vi "Cannon Logic.vi"() -> ()   [LabVIEW 2019]
uses:
  <vilib>/Rock Robotics/WPI/Solenoid/WPI_SolenoidValue.ctl
  <vilib>/Rock Robotics/WPI/ThirdParty/Phoenix-LabVIEW/Motor Controller/Controls/CTRE_Phoenix_MotorControl_ControlMode.ctl
  <vilib>/Rock Robotics/Network Tables/NT Read Boolean.vi
  Robot Global Data.vi
  <vilib>/Rock Robotics/Network Tables/NT Write Number.vi
  <vilib>/Rock Robotics/WPI/Solenoid/WPI_SolenoidSetEnum.vi
panel:
  out "ballcount":i16
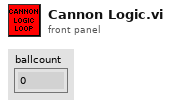
[diagram p1: front panel]
types:
  T1 = typedef "WPI_SolenoidDevRef.ctl" = cluster{"DevStatus":errorcluster, "Pneumatics Control Module":u8, "Forward Solenoid Channel":T2, "Reverse Solenoid Channel":T2}
  T2 = typedef "WPI_SolenoidChannel.ctl" = enum8{"Solenoid 0", "Solenoid 1", "Solenoid 2", "Solenoid 3", "Solenoid 4", "Solenoid 5", "Solenoid 6", "Solenoid 7", "Invalid"}
  T3 = typedef "WPI_MotorControlDeviceRef.ctl" = cluster{"DeviceStatus":errorcluster, "Type":T4, "PWM":cluster{"PWM Channel":T5, "DeadBand":T6}, "CAN":cluster{"Device Number":u8, "SetOutput VI Ref":variant, "GetOutput VI Ref":variant, "Enable VI Ref":variant, "Disable VI Ref":variant, "Data":variant}, "Invert":bool, "DIO PWM":cluster{"PWM \"Enable\" Channel":T5, "DIOChannel":T7, "PWM Rate":dbl}}
  T4 = typedef "WPI_MotorControlType.ctl" = enum16{"PWM", "CAN", "DIO PWM"}
  T5 = typedef "FPGA_DIOPWMChannel.ctl" = enum8{"PWM 0", "PWM 1", "PWM 2", "PWM 3", "PWM 4", "PWM 5", "PWM 6", "PWM 7", "PWM 8", "PWM 9", "PWM MXP 0", "PWM MXP 1", "PWM MXP 2", "PWM MXP 3", "PWM MXP 4", "PWM MXP 5", "PWM MXP 6", "PWM MXP 7", "PWM MXP 8", "PWM MXP 9", "Invalid"}
  T6 = typedef "WPI_PWMDeadband.ctl" = cluster{"Name":string, "maxPositivePwm":i32, "minPositivePwm":i32, "centerPwm":i32, "maxNegativePwm":i32, "minNegativePwm":i32, "angularRange":u16}
  T7 = typedef "FPGA_DIOChannel.ctl" = enum8{"DIO 0", "DIO 1", "DIO 2", "DIO 3", "DIO 4", "DIO 5", "DIO 6", "DIO 7", "DIO 8", "DIO 9", "DIO MXP 0", "DIO MXP 1", "DIO MXP 2", "DIO MXP 3", "DIO MXP 4", "DIO MXP 5", "DIO MXP 6", "DIO MXP 7", "DIO MXP 8", "DIO MXP 9", "DIO MXP 10", "DIO MXP 11", "DIO MXP 12", "DIO MXP 13", "DIO MXP 14", "DIO MXP 15", "SPI Port CS1", "SPI Port CS2", "SPI Port CS3", "SPI Port MISO", "SPI Port MOSI", "Invalid"}
  T8 = typedef "WPI_AnalogChannelDevRef.ctl" = cluster{"DevStatus":errorcluster, "Analog Channel":T9}
  T9 = typedef "FPGA_AIChannel.ctl" = enum8{"AI 0", "AI 1", "AI 2", "AI 3", "AI MXP 0", "AI MXP 1", "AI MXP 2", "AI MXP 3", "Invalid"}
  T10 = typedef "WPI_EncoderDevRef.ctl" = cluster{"DevStatus":errorcluster, "EncoderIndex":T11, "CounterIndex":T12, "DistancePerCount":dbl, "Decoding Type":T13}
  T11 = typedef "FPGA_EncoderIdx.ctl" = enum8{"Enc 0", "Enc 1", "Enc 2", "Enc 3", "Enc 4", "Enc 5", "Enc 6", "Enc 7", "Invalid"}
  T12 = typedef "FPGA_CounterCtrSystemIndex.ctl" = enum8{"Ctr 0", "Ctr 1", "Ctr 2", "Ctr 3", "Ctr 4", "Ctr 5", "Ctr 6", "Ctr 7", "Invalid"}
  T13 = typedef "WPI_EncoderType.ctl" = enum16{"1x", "2x", "4x"}
  T14 = typedef "WPI_SolenoidValue.ctl" = enum16{"Off", "On", "Forward", "Reverse"}
  T15 = typedef "CTRE_Phoenix_MotorControl_ControlMode.ctl" = u16
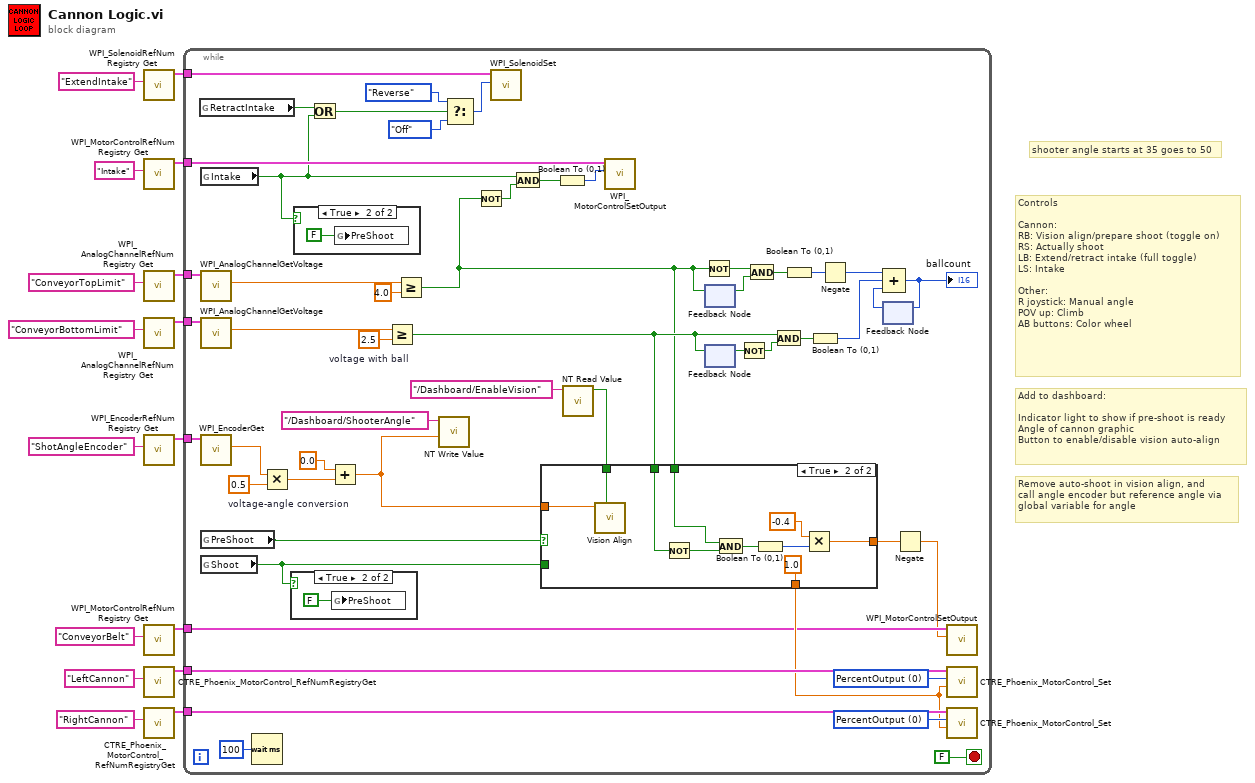
[diagram p0: block diagram]
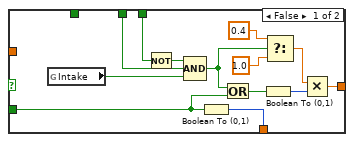
[diagram p4: hidden frame]
diagram:
  # "shooter angle starts at 35 goes to 50"
  # "Remove auto-shoot in vision align, and\ncall angle encoder but reference angle via\nglobal variable for angle"
  # "Add to dashboard:\n\nIndicator light to show if pre-shoot is ready\nAngle of cannon graphic\nButton to enable/disable vision auto-align"
  # "Controls\n\nCannon:\nRB: Vision align/prepare shoot (toggle on)\nRS: Actually shoot\nLB: Extend/retract intake (full toggle)\nLS: Intake\n\nOther:\nR joystick: Manual angle\nPOV up: Climb\nAB buttons: Color wheel"
  n1 = call <vilib>:"WPI_SolenoidRefNum Registry Get.vi"("refnum name"="ExtendIntake") -> ("SolenoidDevRef"=w10:T1)  [unwired: 9 in, 1 out]
  n2 = call <vilib>:"WPI_MotorControlRefNum Registry Get.vi"("refnum name"="Intake") -> ("MotorControlDevRef"=w9:T3)  [unwired: 9 in, 1 out]
  n3 = call <vilib>:"WPI_AnalogChannelRefNum Registry Get.vi"("refnum name"="ConveyorTopLimit") -> ("AIDeviceRef"=w6:T8)  [unwired: 9 in, 1 out]
  n4 = call <vilib>:"WPI_AnalogChannelRefNum Registry Get.vi"("refnum name"="ConveyorBottomLimit") -> ("AIDeviceRef"=w7:T8)  [unwired: 9 in, 1 out]
  n5 = call <vilib>:"WPI_EncoderRefNum Registry Get.vi"("refnum name"="ShotAngleEncoder") -> ("EncoderDevRef"=w1:T10)  [unwired: 9 in, 1 out]
  n6 = call <vilib>:"WPI_MotorControlRefNum Registry Get.vi"("refnum name"="ConveyorBelt") -> ("MotorControlDevRef"=w5:T3)  [unwired: 9 in, 1 out]
  n7 = call <vilib>:"CTRE_Phoenix_MotorControl_RefNumRegistryGet.vi"("refnum name"="LeftCannon") -> ("PhoenixMotorControlDevRef"=w3:T3)  [unwired: 9 in, 1 out]
  n8 = call <vilib>:"CTRE_Phoenix_MotorControl_RefNumRegistryGet.vi"("refnum name"="RightCannon") -> ("PhoenixMotorControlDevRef"=w8:T3)  [unwired: 9 in, 1 out]
  n9 = while {
    tunnel: w10 -> [w63]
    tunnel: w9 -> [w49]
    tunnel: w8 -> [w61]
    tunnel: w7 -> [w60]
    tunnel: w6 -> [w59]
    tunnel: w5 -> [w48]
    tunnel: w3 -> [w55]
    tunnel: w1 -> [w21]
    stop <- FALSE stop-if-true
    w22 = 0.5  # voltage-angle conversion
    w56 = T15 0 items=["PercentOutput"=0, "Position"=1, "Velocity"=2, "Current"=3, "Follower"=5, "MotionProfile"=6, "MotionMagic"=7, "MotionProfileArc"=10, "Disabled"=15] ("Control Mode")
    w54 = T15 0 items=["PercentOutput"=0, "Position"=1, "Velocity"=2, "Current"=3, "Follower"=5, "MotionProfile"=6, "MotionMagic"=7, "MotionProfileArc"=10, "Disabled"=15] ("Control Mode")
    w57 = 2.5  # voltage with ball
    n10 = global read "Robot Global Data.vi" "RetractIntake"() -> (w35:bool)
    n11 = global read "Robot Global Data.vi" "Intake"() -> (w28:bool)
    n12 = call <vilib>:"WPI_AnalogChannelGetVoltage.vi"("AIDeviceRef"=w59) -> ("Voltage"=w30:dbl)  [unwired: 8 in, 2 out]
    n13 = call <vilib>:"WPI_AnalogChannelGetVoltage.vi"("AIDeviceRef"=w60) -> ("Voltage"=w29:dbl)  [unwired: 8 in, 2 out]
    n14 = call <vilib>:"WPI_EncoderGet.vi"("EncoderDevRef"=w21) -> ("Distance"=w23:dbl)  [unwired: 5 in, 5 out]
    n15 = global read "Robot Global Data.vi" "PreShoot"() -> (w33:bool)
    n16 = global read "Robot Global Data.vi" "Shoot"() -> (w34:bool)
    n17 = Wait (ms)(milliseconds to wait=u32 100) -> ()  [unwired: 1 out]
    n18 = Multiply(x=w23, y=w22) -> (x*y=w19:dbl)
    n19 = case shown="True" w34 {
      frame False {
      }
      frame True {
        n20 = global write "Robot Global Data.vi" "PreShoot"(FALSE ("PreShoot")) -> ()
      }
    }
    n21 = case shown="True" w28 {
      frame False {
      }
      frame True {
        n22 = global write "Robot Global Data.vi" "PreShoot"(FALSE ("PreShoot")) -> ()
      }
    }
    n23 = Or(x=w35, y=w28) -> (x .or. y?=w66:bool)
    n24 = Add(x=0.0, y=w19) -> (x+y=w18:dbl)
    n25 = Greater Or Equal?(x=w29, y=w57) -> (x >= y?=w25:bool)
    n26 = Greater Or Equal?(x=w30, y=4.0) -> (x >= y?=w24:bool)
    n27 = call-poly <vilib>:"NT Write Value.vi"("Numeric"=w18, "Name"="/Dashboard/ShooterAngle") -> ()  [unwired: 9 in, 1 out]
    n28 = Select(t=WPI_SolenoidValue."Reverse" ("Value"), s=w66, f=WPI_SolenoidValue."Off" ("Value")) -> (s? t:f=w62:T14)
    n29 = Not(x=w24) -> (.not. x?=w26:bool)
    n30 = call-poly <vilib>:"WPI_SolenoidSet.vi"("Value"=w62, "SolenoidDevRef"=w63) -> ()  [unwired: 8 in, 2 out]
    n31 = And(x=w28, y=w26) -> (x .and. y?=w27:bool)
    n32 = Boolean To (0,1)(Boolean=w27) -> (0, 1=w58:i16)
    n33 = call-poly <vilib>:"NT Read Value.vi"("Name"="/Dashboard/EnableVision") -> ("Boolean"=w47:bool)  [unwired: 9 in, 1 out]
    n34 = case shown="True" w33 {
      tunnel: [w80 w85] -> w31
      tunnel: [w79 1.0] -> w50
      tunnel: w34 -> [w71 _]
      tunnel: w24 -> [w72 w87]
      tunnel: w47 -> [_ w83]
      tunnel: w25 -> [w81 w88]
      tunnel: w18 -> [_ w84]
      frame False {
        n35 = global read "Robot Global Data.vi" "Intake"() -> (w78:bool)
        n36 = Not(x=w72) -> (.not. x?=w70:bool)
        n37 = Compound Arithmetic op=AND(w70, w81, w78) -> (w76:bool)
        n38 = Boolean To (0,1)(Boolean=w71) -> (0, 1=w79:i16)
        n39 = Or(x=w76, y=w71) -> (x .or. y?=w82:bool)
        n40 = Boolean To (0,1)(Boolean=w82) -> (0, 1=w74:i16)
        n41 = Select(t=0.4, s=w76, f=1.0) -> (s? t:f=w73:dbl)
        n42 = Multiply(x=w73, y=w74) -> (x*y=w80:dbl)
      }
      frame True {
        n43 = call "Vision Align.vi"("VisionEnabled"=w83, "AngleEncoder"=w84) -> ()  [unwired: 10 in]
        n44 = Not(x=w88) -> (.not. x?=w86:bool)
        n45 = And(x=w87, y=w86) -> (x .and. y?=w90:bool)
        n46 = Boolean To (0,1)(Boolean=w90) -> (0, 1=w91:i16)
        n47 = Multiply(x=-0.4, y=w91) -> (x*y=w85:dbl)
      }
    }
    n48 = call <vilib>:"WPI_MotorControlSetOutput.vi"("Output"=w58, "MotorControlDevRef"=w49) -> ()  [unwired: 7 in, 3 out]
    n49 = Not(x=w24) -> (.not. x?=w46:bool)
    n50 = feedback-in #1(w24) -> ()
    n51 = feedback #1() -> (w45:bool)  [unwired: 1 in]
    n52 = feedback #2() -> (w44:bool)  [unwired: 1 in]
    n53 = feedback-in #2(w25) -> ()
    n54 = Not(x=w44) -> (.not. x?=w43:bool)
    n55 = And(x=w46, y=w45) -> (x .and. y?=w42:bool)
    n56 = And(x=w25, y=w43) -> (x .and. y?=w41:bool)
    n57 = Boolean To (0,1)(Boolean=w42) -> (0, 1=w40:i16)
    n58 = Boolean To (0,1)(Boolean=w41) -> (0, 1=w36:i16)
    n59 = Negate(x=w40) -> (-x=w39:i16)
    n60 = feedback #3() -> (w38:i16)  [unwired: 1 in]
    n61 = Compound Arithmetic op=ADD(w39, w36, w38) -> (w37:i16)
    "ballcount" <- w37
    n62 = feedback-in #3(w37) -> ()
    n63 = Negate(x=w31) -> (-x=w32:dbl)
    n64 = call <vilib>:"WPI_MotorControlSetOutput.vi"("Output"=w32, "MotorControlDevRef"=w48) -> ()  [unwired: 7 in, 3 out]
    n65 = call <vilib>:"CTRE_Phoenix_MotorControl_Set.vi"("Output"=w50, "Control Mode"=w56, "PhoenixMotorControlDevRef"=w55) -> ()  [unwired: 7 in, 2 out]
    n66 = call <vilib>:"CTRE_Phoenix_MotorControl_Set.vi"("Output"=w50, "Control Mode"=w54, "PhoenixMotorControlDevRef"=w61) -> ()  [unwired: 7 in, 2 out]
  }
